vi "Alinhamento.vi"() -> ()   [LabVIEW 2019]
uses:
  <vilib>/silver_ctls/ArrayMatrixCluster/Real Matrix NI_Silver.ctl
panel:
  in  "MWU2987":i16
  in  "MWU2986":i16
  in  "MWU2985":i16
  in  "MWU2984":i16
  in  "MWU2983":i16
  in  "MWU2982":i16
  in  "MWU2981":i16
  in  "MWU2980":i16
  in  "MWU2979":i16
  in  "MWU2978":i16
  in  "MWU2977":i16
  in  "MWU2976":i16
  in  "MWU2975":i16
  in  "Tab Control":enum32{"Gráfico", "Matriz"}(tab)
  out "MWU1100":i16
  out "String lida em Caracter":string
  out "Gráfico":cluster{dbl, dbl, "Real Matrix":dbl[][]}(graph)
  out "Tubo":dbl(slide) scale=0.0..1950.0
  in  "Iniciar":bool
  in  "Parar":bool
  out "appended array":T1
  # "Valor enviado para a \ncomunicação"
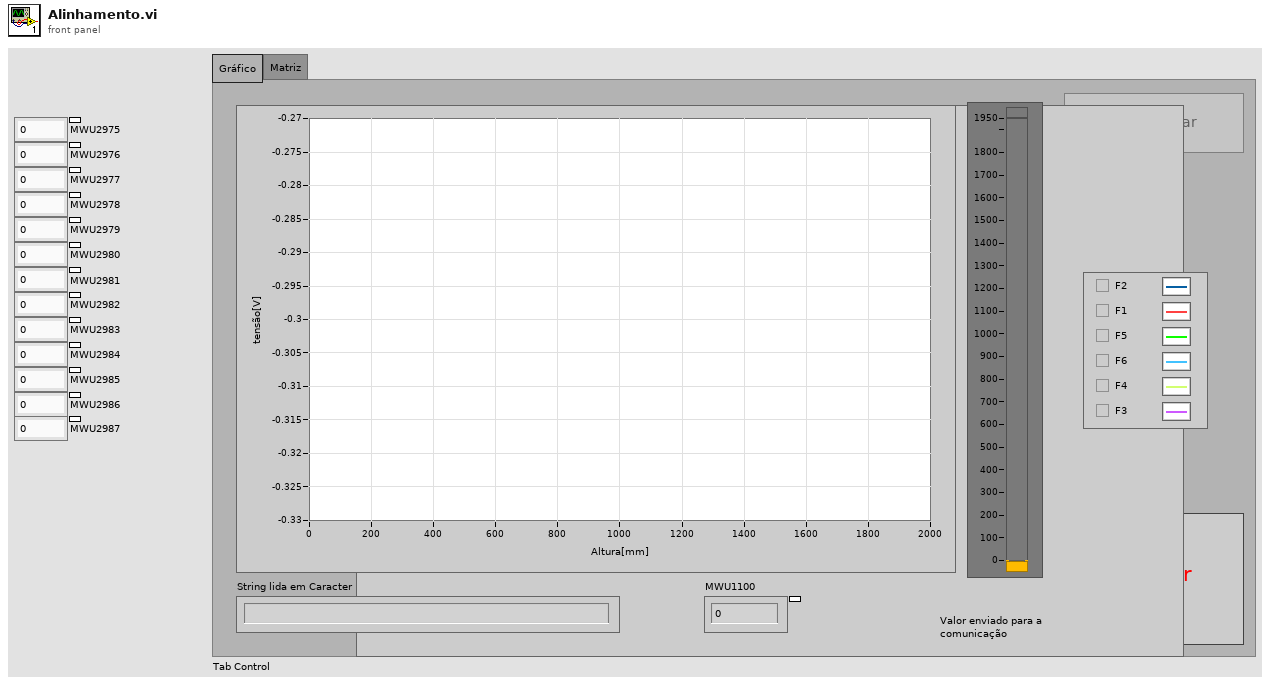
[diagram p1: front panel]
types:
  T1 = typedef "Real Matrix NI_Silver.ctl" = dbl[][]
  T2 = enum8{"Enabled", "Disabled", "Disabled and Grayed Out"}
  T3 = typedef "NI_Matrix.lvlib/RealMatrix.ctl" = dbl[][]
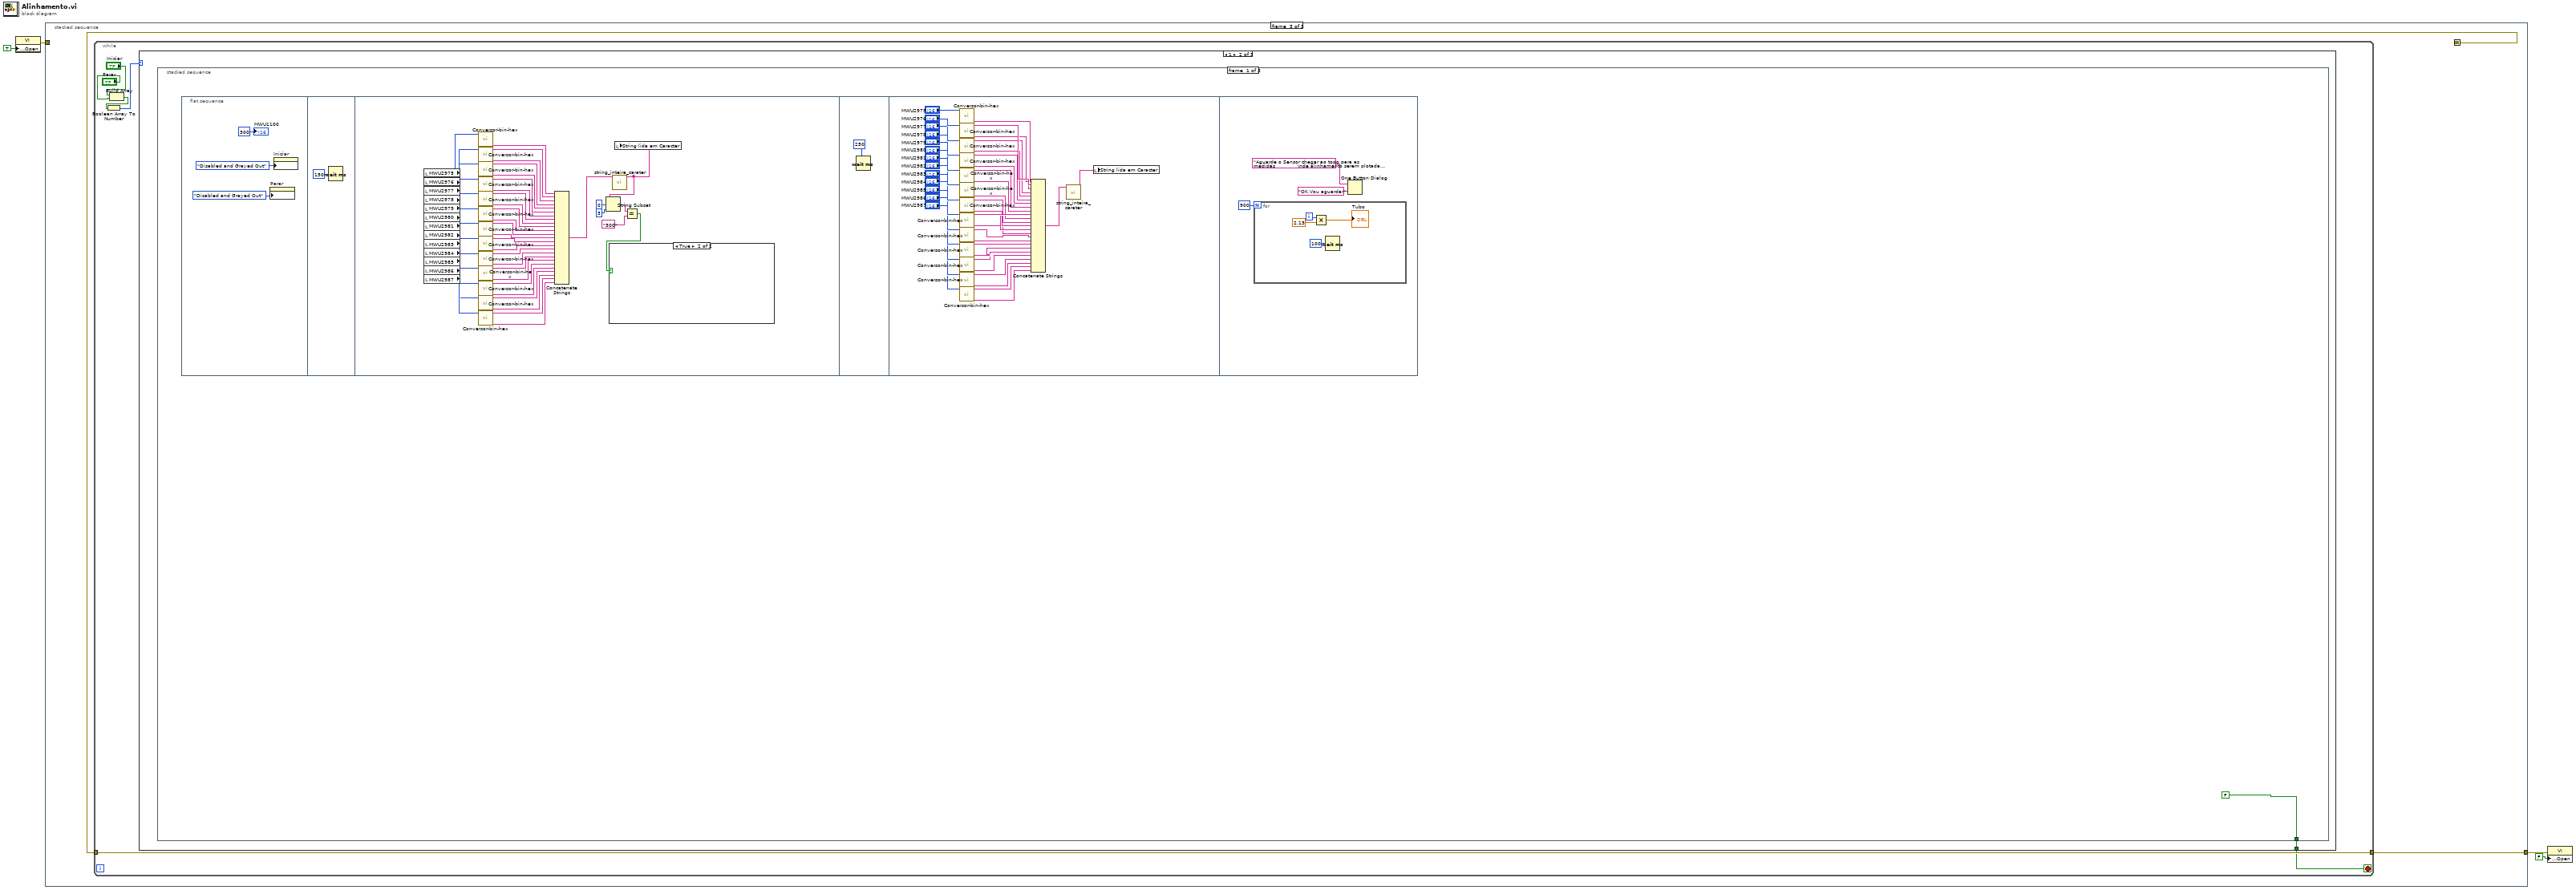
[diagram p0: block diagram]
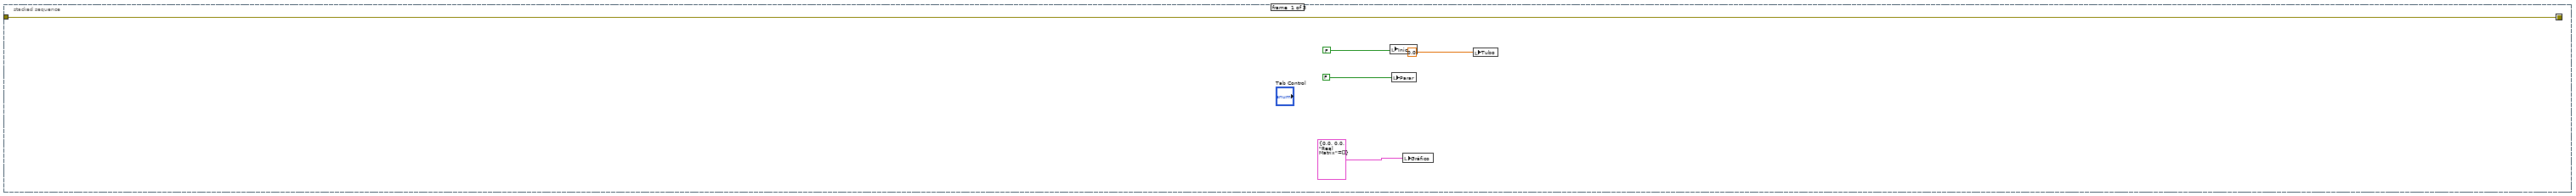
[diagram p2: hidden frame]
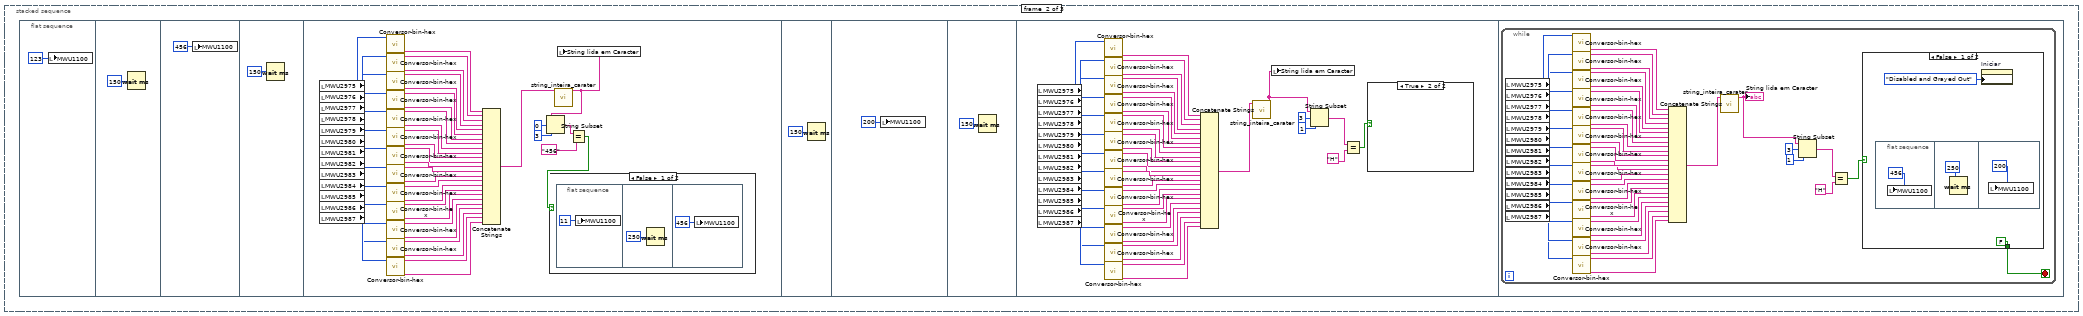
[diagram p3: hidden frame]
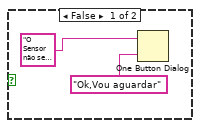
[diagram p5: hidden frame]
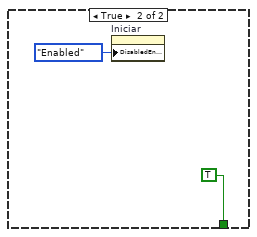
[diagram p6: hidden frame]
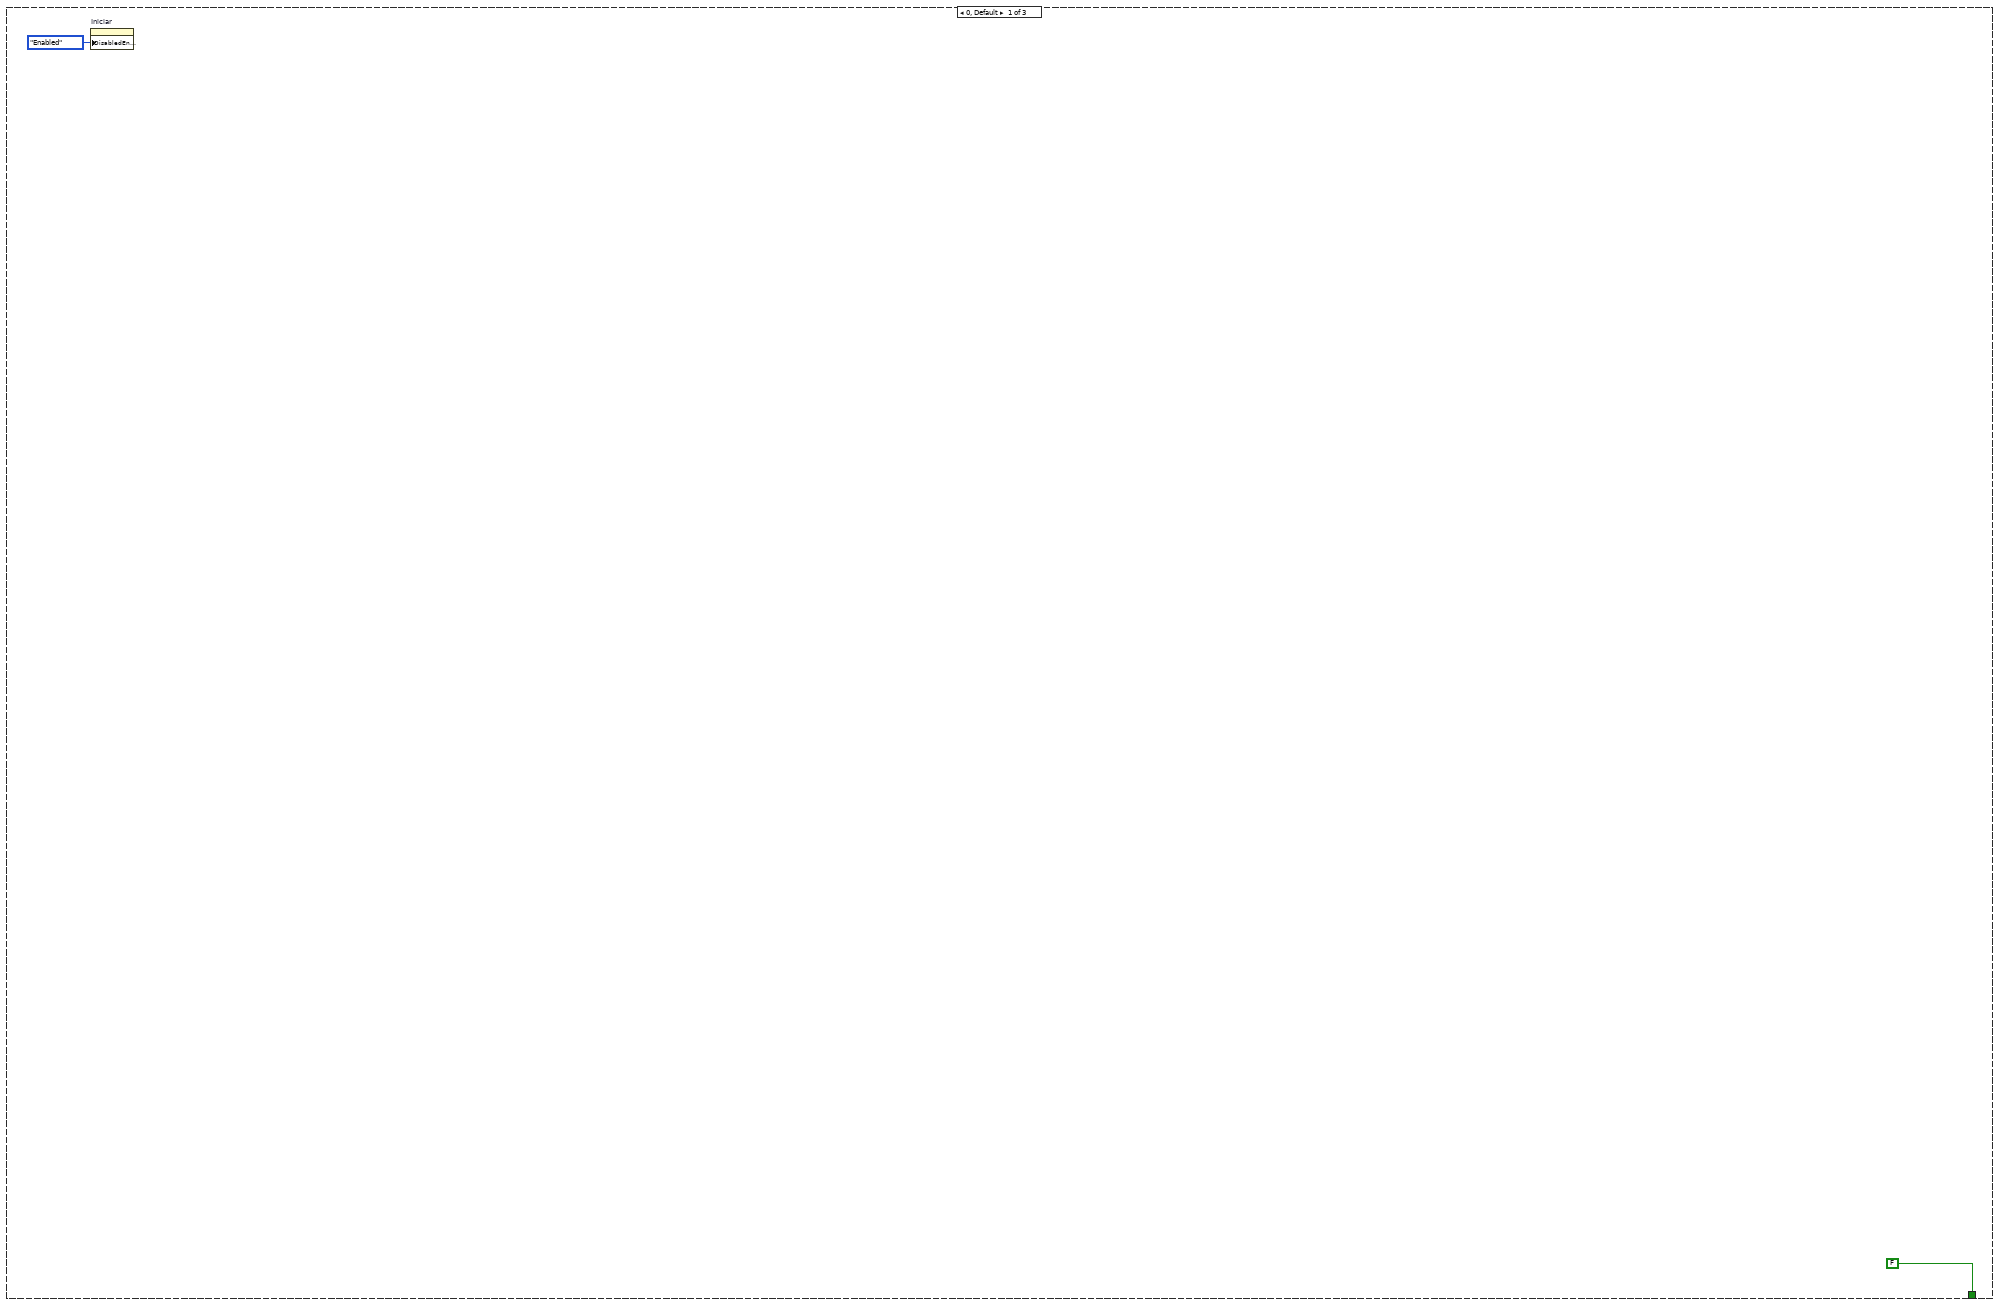
[diagram p7: hidden frame]
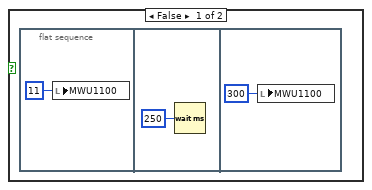
[diagram p8: hidden frame]
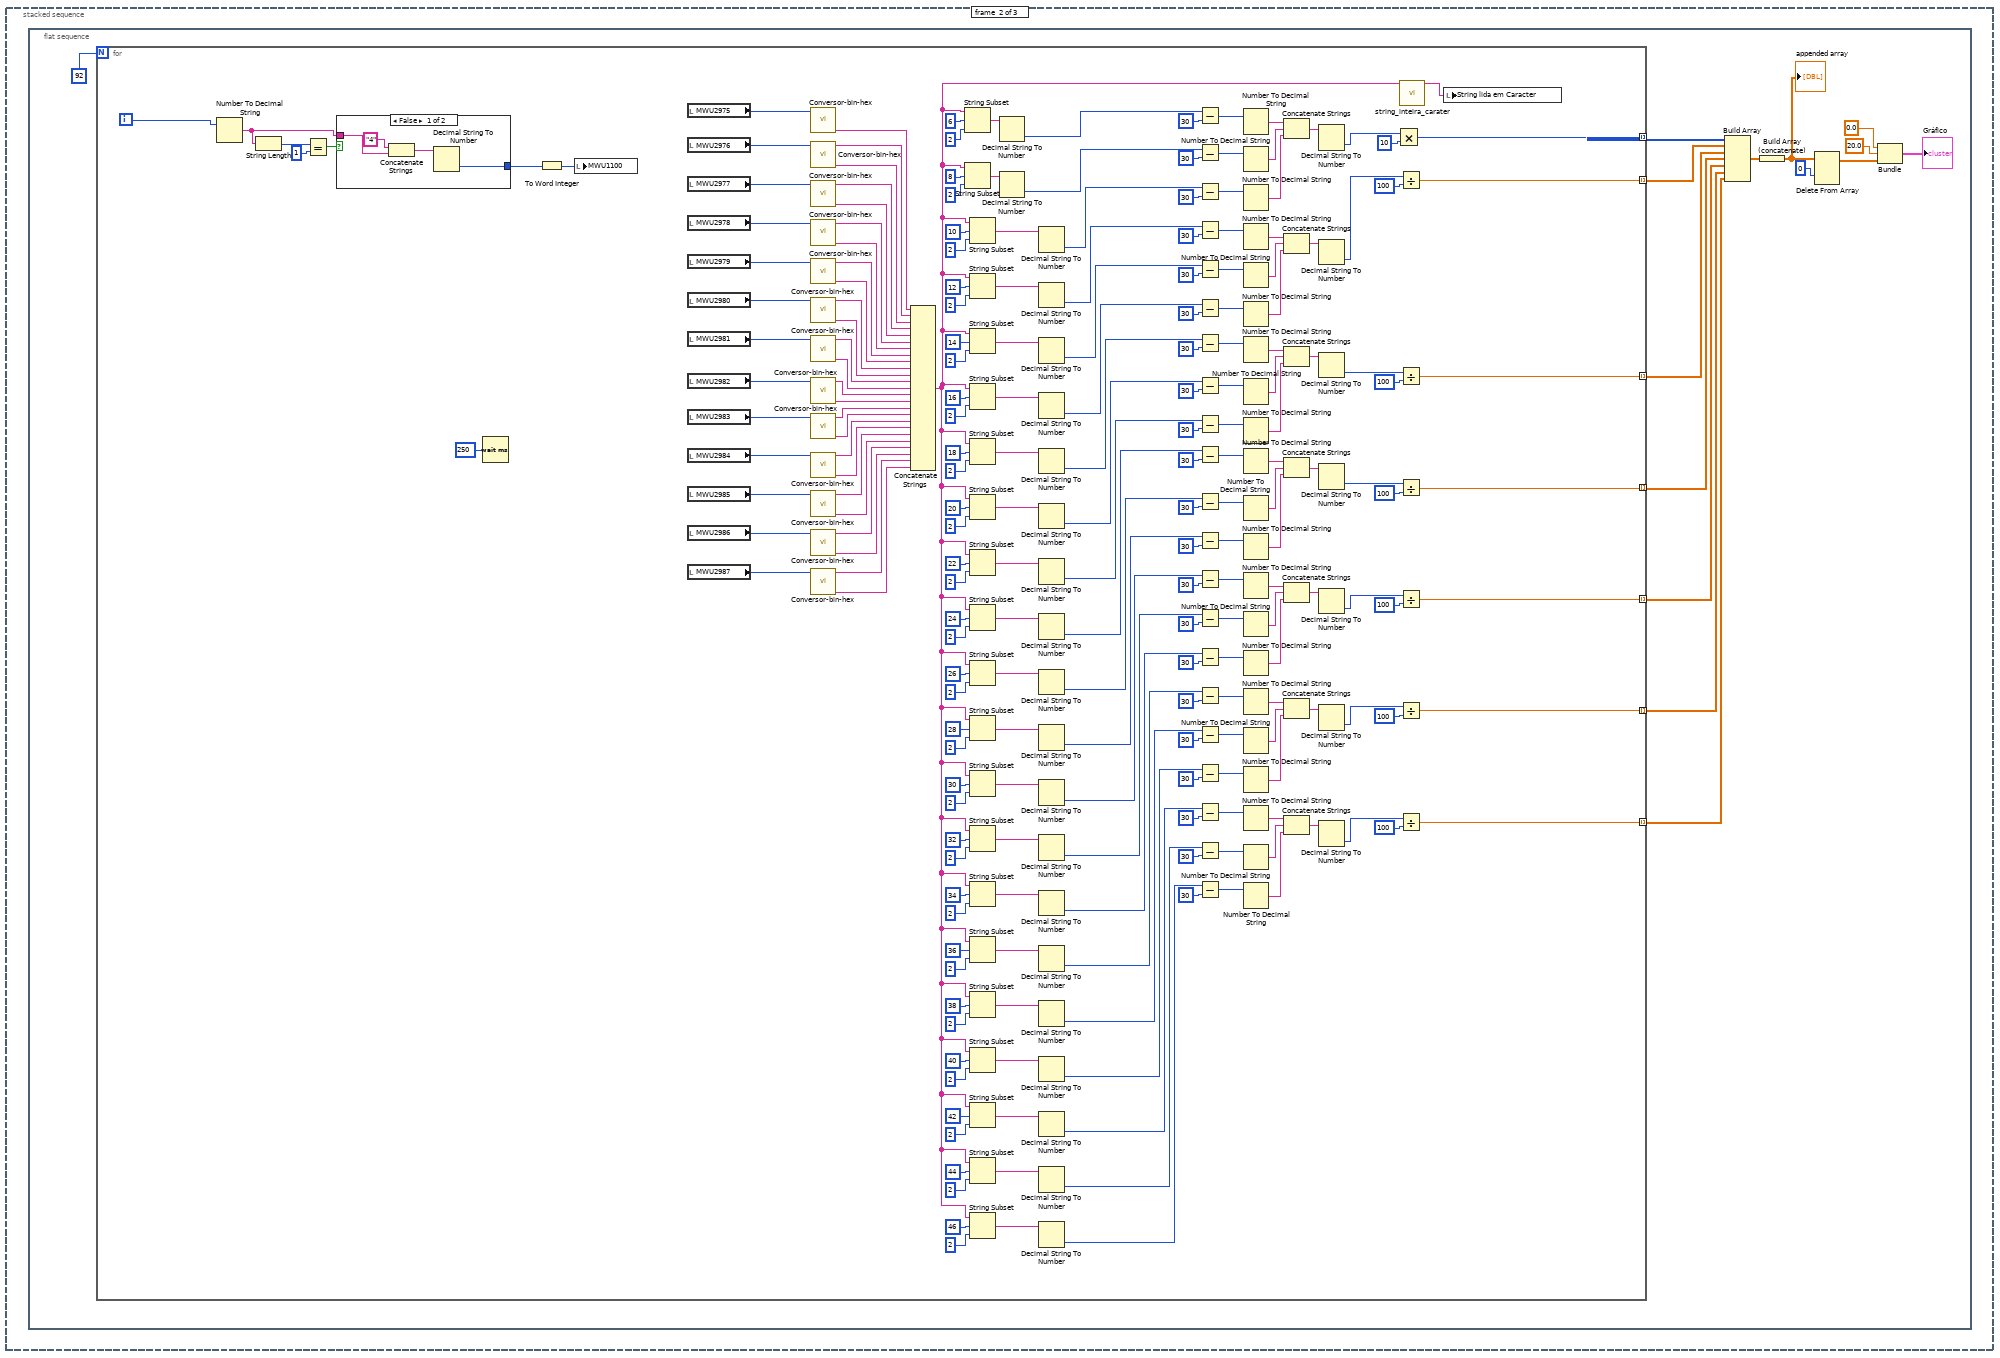
[diagram p9: hidden frame]
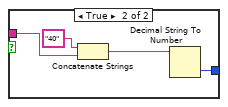
[diagram p10: hidden frame]
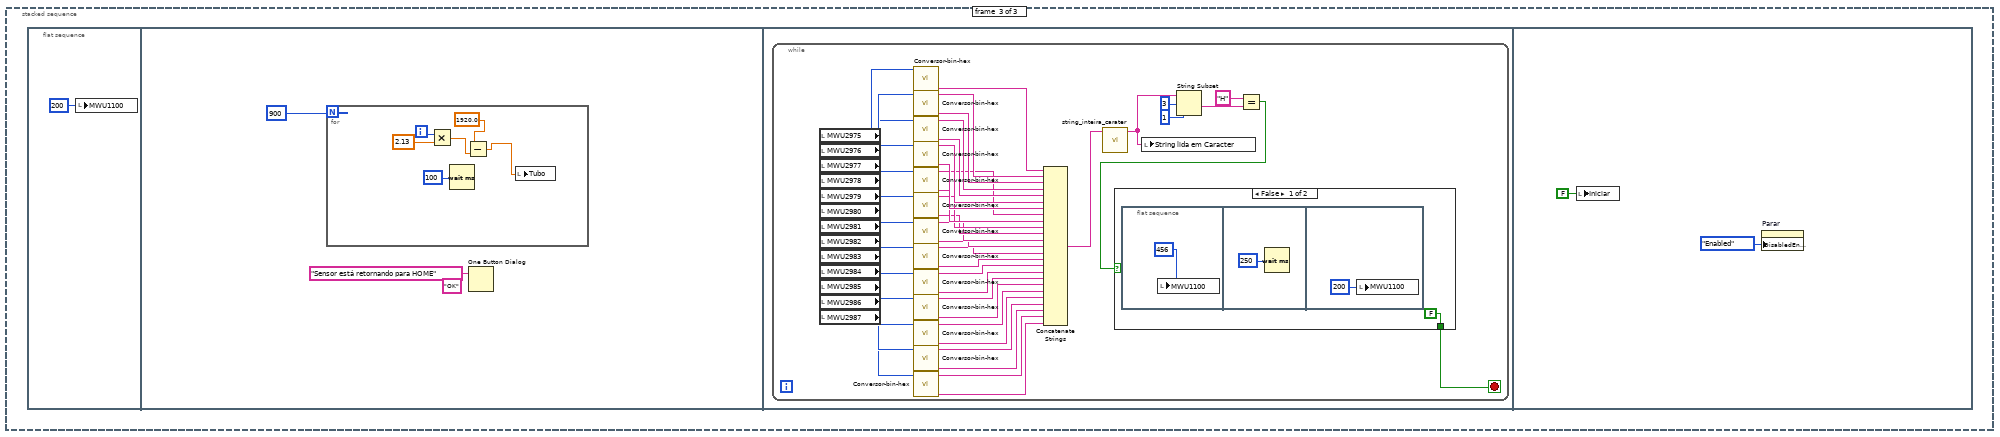
[diagram p11: hidden frame]
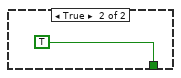
[diagram p12: hidden frame]
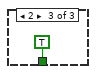
[diagram p13: hidden frame]
diagram:
  n1 = property class="VI"("Front Panel.Open"=TRUE ("Front Panel Window:Open")) -> (error out=w2:errorcluster)  [unwired: 2 in, 1 out]
  n2 = stacked-sequence {
    seq-local: [w9 _ _] -> [_ _ w166]
    tunnel: w2 -> [w9 _ _]
    tunnel: [_ _ w165] -> w1
    frame #0 {
      n3 = local write "Iniciar"(FALSE ("Iniciar")) -> ()
      n4 = local write "Parar"(FALSE ("Parar")) -> ()
      n5 = local write "Gráfico"(cluster{dbl, dbl, "Real Matrix":dbl[][]} {0.0, 0.0, "Real Matrix"=[]} ("Gráfico")) -> ()
      n6 = local write "Tubo"(0.0 ("Tubo")) -> ()
    }
    frame #1 {
      n7 = flat-sequence {
        frame #0 {
          n8 = local write "MWU1100"(i16 123 ("MWU1100")) -> ()
        }
        frame #1 {
          n9 = Wait (ms)(milliseconds to wait=u32 150) -> ()  [unwired: 1 out]
        }
        frame #2 {
          n10 = local write "MWU1100"(i16 456 ("MWU1100")) -> ()
        }
        frame #3 {
          n11 = Wait (ms)(milliseconds to wait=u32 150) -> ()  [unwired: 1 out]
        }
        frame #4 {
          n12 = local read "MWU2975"() -> (w44:i16)
          n13 = local read "MWU2976"() -> (w45:i16)
          n14 = local read "MWU2977"() -> (w46:i16)
          n15 = local read "MWU2978"() -> (w47:i16)
          n16 = local read "MWU2979"() -> (w48:i16)
          n17 = local read "MWU2980"() -> (w49:i16)
          n18 = local read "MWU2981"() -> (w50:i16)
          n19 = local read "MWU2982"() -> (w51:i16)
          n20 = local read "MWU2983"() -> (w52:i16)
          n21 = local read "MWU2984"() -> (w53:i16)
          n22 = local read "MWU2985"() -> (w54:i16)
          n23 = local read "MWU2986"() -> (w55:i16)
          n24 = local read "MWU2987"() -> (w56:i16)
          n25 = call "Conversor-bin-hex.vi"("Numeric"=w44) -> ("hex integer string"=w20:string)  [unwired: 9 in, 1 out]
          n26 = call "Conversor-bin-hex.vi"("Numeric"=w45) -> ("hex integer string"=w22:string, "hex integer string 2"=w21:string)  [unwired: 9 in]
          n27 = call "Conversor-bin-hex.vi"("Numeric"=w46) -> ("hex integer string"=w24:string, "hex integer string 2"=w23:string)  [unwired: 9 in]
          n28 = call "Conversor-bin-hex.vi"("Numeric"=w47) -> ("hex integer string"=w26:string, "hex integer string 2"=w25:string)  [unwired: 9 in]
          n29 = call "Conversor-bin-hex.vi"("Numeric"=w48) -> ("hex integer string"=w28:string, "hex integer string 2"=w27:string)  [unwired: 9 in]
          n30 = call "Conversor-bin-hex.vi"("Numeric"=w49) -> ("hex integer string"=w30:string, "hex integer string 2"=w29:string)  [unwired: 9 in]
          n31 = call "Conversor-bin-hex.vi"("Numeric"=w50) -> ("hex integer string"=w32:string, "hex integer string 2"=w31:string)  [unwired: 9 in]
          n32 = call "Conversor-bin-hex.vi"("Numeric"=w51) -> ("hex integer string"=w34:string, "hex integer string 2"=w33:string)  [unwired: 9 in]
          n33 = call "Conversor-bin-hex.vi"("Numeric"=w52) -> ("hex integer string"=w36:string, "hex integer string 2"=w35:string)  [unwired: 9 in]
          n34 = call "Conversor-bin-hex.vi"("Numeric"=w53) -> ("hex integer string"=w38:string, "hex integer string 2"=w37:string)  [unwired: 9 in]
          n35 = call "Conversor-bin-hex.vi"("Numeric"=w54) -> ("hex integer string"=w40:string, "hex integer string 2"=w39:string)  [unwired: 9 in]
          n36 = call "Conversor-bin-hex.vi"("Numeric"=w55) -> ("hex integer string"=w42:string, "hex integer string 2"=w41:string)  [unwired: 9 in]
          n37 = call "Conversor-bin-hex.vi"("Numeric"=w56) -> ("hex integer string"=w57:string, "hex integer string 2"=w43:string)  [unwired: 9 in]
          n38 = Concatenate Strings(w20, w21, w22, w23, w24, w25, w26, w27, w28, w29, w30, w31, w32, w33, w34, w35, w36, w37, w38, w39, w40, w41, w42, w43, w57) -> (w58:string)
          n39 = call "string_inteira_carater.vi"("String in"=w58) -> ("String out"=w19:string)  [unwired: 10 in]
          n40 = String Subset(string=w19, offset (0)=0, length (rest)=3 ("length (rest)")) -> (substring=w16:string)
          n41 = local write "String lida em Caracter"(w19) -> ()
          n42 = Equal?(x=w16, y="456") -> (x = y?=w14:bool)
          n43 = case shown="False" w14 {
            frame False {
              n44 = flat-sequence {
                frame #0 {
                  n45 = local write "MWU1100"(i16 11 ("MWU1100")) -> ()
                }
                frame #1 {
                  n46 = Wait (ms)(milliseconds to wait=u32 250) -> ()  [unwired: 1 out]
                }
                frame #2 {
                  n47 = local write "MWU1100"(i16 456 ("MWU1100")) -> ()
                }
              }
            }
            frame True {
            }
          }
        }
        frame #5 {
          n48 = Wait (ms)(milliseconds to wait=u32 150) -> ()  [unwired: 1 out]
        }
        frame #6 {
          n49 = local write "MWU1100"(i16 200 ("MWU1100")) -> ()
        }
        frame #7 {
          n50 = Wait (ms)(milliseconds to wait=u32 150) -> ()  [unwired: 1 out]
        }
        frame #8 {
          n51 = local read "MWU2975"() -> (w71:i16)
          n52 = local read "MWU2976"() -> (w96:i16)
          n53 = local read "MWU2977"() -> (w97:i16)
          n54 = local read "MWU2978"() -> (w98:i16)
          n55 = local read "MWU2979"() -> (w99:i16)
          n56 = local read "MWU2980"() -> (w100:i16)
          n57 = local read "MWU2981"() -> (w101:i16)
          n58 = local read "MWU2982"() -> (w102:i16)
          n59 = local read "MWU2983"() -> (w103:i16)
          n60 = local read "MWU2984"() -> (w104:i16)
          n61 = local read "MWU2985"() -> (w105:i16)
          n62 = local read "MWU2986"() -> (w106:i16)
          n63 = local read "MWU2987"() -> (w107:i16)
          n64 = call "Conversor-bin-hex.vi"("Numeric"=w71) -> ("hex integer string"=w72:string)  [unwired: 9 in, 1 out]
          n65 = call "Conversor-bin-hex.vi"("Numeric"=w96) -> ("hex integer string"=w74:string, "hex integer string 2"=w73:string)  [unwired: 9 in]
          n66 = call "Conversor-bin-hex.vi"("Numeric"=w97) -> ("hex integer string"=w76:string, "hex integer string 2"=w75:string)  [unwired: 9 in]
          n67 = call "Conversor-bin-hex.vi"("Numeric"=w98) -> ("hex integer string"=w78:string, "hex integer string 2"=w77:string)  [unwired: 9 in]
          n68 = call "Conversor-bin-hex.vi"("Numeric"=w99) -> ("hex integer string"=w80:string, "hex integer string 2"=w79:string)  [unwired: 9 in]
          n69 = call "Conversor-bin-hex.vi"("Numeric"=w100) -> ("hex integer string"=w82:string, "hex integer string 2"=w81:string)  [unwired: 9 in]
          n70 = call "Conversor-bin-hex.vi"("Numeric"=w101) -> ("hex integer string"=w84:string, "hex integer string 2"=w83:string)  [unwired: 9 in]
          n71 = call "Conversor-bin-hex.vi"("Numeric"=w102) -> ("hex integer string"=w86:string, "hex integer string 2"=w85:string)  [unwired: 9 in]
          n72 = call "Conversor-bin-hex.vi"("Numeric"=w103) -> ("hex integer string"=w88:string, "hex integer string 2"=w87:string)  [unwired: 9 in]
          n73 = call "Conversor-bin-hex.vi"("Numeric"=w104) -> ("hex integer string"=w90:string, "hex integer string 2"=w89:string)  [unwired: 9 in]
          n74 = call "Conversor-bin-hex.vi"("Numeric"=w105) -> ("hex integer string"=w92:string, "hex integer string 2"=w91:string)  [unwired: 9 in]
          n75 = call "Conversor-bin-hex.vi"("Numeric"=w106) -> ("hex integer string"=w94:string, "hex integer string 2"=w93:string)  [unwired: 9 in]
          n76 = call "Conversor-bin-hex.vi"("Numeric"=w107) -> ("hex integer string"=w108:string, "hex integer string 2"=w95:string)  [unwired: 9 in]
          n77 = Concatenate Strings(w72, w73, w74, w75, w76, w77, w78, w79, w80, w81, w82, w83, w84, w85, w86, w87, w88, w89, w90, w91, w92, w93, w94, w95, w108) -> (w109:string)
          n78 = call "string_inteira_carater.vi"("String in"=w109) -> ("String out"=w66:string)  [unwired: 10 in]
          n79 = local write "String lida em Caracter"(w66) -> ()
          n80 = String Subset(string=w66, offset (0)=3, length (rest)=1 ("length (rest)")) -> (substring=w67:string)
          n81 = Equal?(x=w67, y="H") -> (x = y?=w65:bool)
          n82 = case shown="True" w65 {
            frame False {
              n83 = One Button Dialog(message="O Sensor não se encontra em HOME                          \nEle já está descendo, aguarde chegar para começar o alinhamento", button name ("OK")="Ok,Vou aguardar") -> ()  [unwired: 1 out]
            }
            frame True {
            }
          }
        }
        frame #9 {
          n84 = while {
            stop <- w113 stop-if-true
            n85 = local read "MWU2975"() -> (w133:i16)
            n86 = local read "MWU2976"() -> (w132:i16)
            n87 = local read "MWU2977"() -> (w131:i16)
            n88 = local read "MWU2978"() -> (w130:i16)
            n89 = local read "MWU2979"() -> (w129:i16)
            n90 = local read "MWU2980"() -> (w128:i16)
            n91 = local read "MWU2981"() -> (w127:i16)
            n92 = local read "MWU2982"() -> (w126:i16)
            n93 = local read "MWU2983"() -> (w125:i16)
            n94 = local read "MWU2984"() -> (w124:i16)
            n95 = local read "MWU2985"() -> (w123:i16)
            n96 = local read "MWU2986"() -> (w122:i16)
            n97 = local read "MWU2987"() -> (w121:i16)
            n98 = call "Conversor-bin-hex.vi"("Numeric"=w133) -> ("hex integer string"=w157:string)  [unwired: 9 in, 1 out]
            n99 = call "Conversor-bin-hex.vi"("Numeric"=w132) -> ("hex integer string"=w155:string, "hex integer string 2"=w156:string)  [unwired: 9 in]
            n100 = call "Conversor-bin-hex.vi"("Numeric"=w131) -> ("hex integer string"=w153:string, "hex integer string 2"=w154:string)  [unwired: 9 in]
            n101 = call "Conversor-bin-hex.vi"("Numeric"=w130) -> ("hex integer string"=w151:string, "hex integer string 2"=w152:string)  [unwired: 9 in]
            n102 = call "Conversor-bin-hex.vi"("Numeric"=w129) -> ("hex integer string"=w149:string, "hex integer string 2"=w150:string)  [unwired: 9 in]
            n103 = call "Conversor-bin-hex.vi"("Numeric"=w128) -> ("hex integer string"=w147:string, "hex integer string 2"=w148:string)  [unwired: 9 in]
            n104 = call "Conversor-bin-hex.vi"("Numeric"=w127) -> ("hex integer string"=w145:string, "hex integer string 2"=w146:string)  [unwired: 9 in]
            n105 = call "Conversor-bin-hex.vi"("Numeric"=w126) -> ("hex integer string"=w143:string, "hex integer string 2"=w144:string)  [unwired: 9 in]
            n106 = call "Conversor-bin-hex.vi"("Numeric"=w125) -> ("hex integer string"=w141:string, "hex integer string 2"=w142:string)  [unwired: 9 in]
            n107 = call "Conversor-bin-hex.vi"("Numeric"=w124) -> ("hex integer string"=w139:string, "hex integer string 2"=w140:string)  [unwired: 9 in]
            n108 = call "Conversor-bin-hex.vi"("Numeric"=w123) -> ("hex integer string"=w137:string, "hex integer string 2"=w138:string)  [unwired: 9 in]
            n109 = call "Conversor-bin-hex.vi"("Numeric"=w122) -> ("hex integer string"=w135:string, "hex integer string 2"=w136:string)  [unwired: 9 in]
            n110 = call "Conversor-bin-hex.vi"("Numeric"=w121) -> ("hex integer string"=w120:string, "hex integer string 2"=w134:string)  [unwired: 9 in]
            n111 = Concatenate Strings(w157, w156, w155, w154, w153, w152, w151, w150, w149, w148, w147, w146, w145, w144, w143, w142, w141, w140, w139, w138, w137, w136, w135, w134, w120) -> (w115:string)
            n112 = call "string_inteira_carater.vi"("String in"=w115) -> ("String out"=w114:string)  [unwired: 10 in]
            "String lida em Caracter" <- w114
            n113 = String Subset(string=w114, offset (0)=3, length (rest)=1 ("length (rest)")) -> (substring=w116:string)
            n114 = Equal?(x=w116, y="H") -> (x = y?=w112:bool)
            n115 = case shown="False" w112 {
              tunnel: [FALSE TRUE] -> w113
              frame False {
                n116 = flat-sequence {
                  frame #0 {
                    n117 = local write "MWU1100"(i16 456 ("MWU1100")) -> ()
                  }
                  frame #1 {
                    n118 = Wait (ms)(milliseconds to wait=u32 250) -> ()  [unwired: 1 out]
                  }
                  frame #2 {
                    n119 = local write "MWU1100"(i16 200 ("MWU1100")) -> ()
                  }
                }
                n120 = property on="Iniciar" class="Bool (strict)"("DisabledEnum"=T2."Disabled and Grayed Out" ("Disabled")) -> ()  [unwired: 2 in, 2 out]
              }
              frame True {
                n121 = property on="Iniciar" class="Bool (strict)"("DisabledEnum"=T2."Enabled" ("Disabled")) -> ()  [unwired: 2 in, 2 out]
              }
            }
          }
        }
      }
    }
    frame #2 {
      n122 = while {
        tunnel: w166 -> [w172]
        tunnel: [w172] -> w165
        stop <- w168 stop-if-true
        n123 = Build Array("Iniciar", "Parar") -> (w170:bool[])
        n124 = Boolean Array To Number(Boolean array=w170) -> (number=w169:u32)
        n125 = case shown="1" w169 {
          tunnel: [FALSE w175 TRUE] -> w168
          frame 0, Default {
            n126 = property on="Iniciar" class="Bool (strict)"("DisabledEnum"=T2."Enabled" ("Disabled")) -> ()  [unwired: 2 in, 2 out]
          }
          frame 1 {
            n127 = stacked-sequence {
              tunnel: [FALSE _ _] -> w175
              frame #0 {
                n128 = flat-sequence {
                  frame #0 {
                    n129 = property on="Parar" class="Bool (strict)"("DisabledEnum"=T2."Disabled and Grayed Out" ("Disabled")) -> ()  [unwired: 2 in, 2 out]
                    n130 = property on="Iniciar" class="Bool (strict)"("DisabledEnum"=T2."Disabled and Grayed Out" ("Disabled")) -> ()  [unwired: 2 in, 2 out]
                    "MWU1100" <- i16 300 ("MWU1100")
                  }
                  frame #1 {
                    n131 = Wait (ms)(milliseconds to wait=u32 150) -> ()  [unwired: 1 out]
                  }
                  frame #2 {
                    n132 = local read "MWU2975"() -> (w211:i16)
                    n133 = local read "MWU2976"() -> (w212:i16)
                    n134 = local read "MWU2977"() -> (w213:i16)
                    n135 = local read "MWU2978"() -> (w214:i16)
                    n136 = local read "MWU2979"() -> (w215:i16)
                    n137 = local read "MWU2980"() -> (w216:i16)
                    n138 = local read "MWU2981"() -> (w217:i16)
                    n139 = local read "MWU2982"() -> (w218:i16)
                    n140 = local read "MWU2983"() -> (w219:i16)
                    n141 = local read "MWU2984"() -> (w220:i16)
                    n142 = local read "MWU2985"() -> (w221:i16)
                    n143 = local read "MWU2986"() -> (w222:i16)
                    n144 = local read "MWU2987"() -> (w223:i16)
                    n145 = call "Conversor-bin-hex.vi"("Numeric"=w211) -> ("hex integer string"=w187:string)  [unwired: 9 in, 1 out]
                    n146 = call "Conversor-bin-hex.vi"("Numeric"=w212) -> ("hex integer string"=w189:string, "hex integer string 2"=w188:string)  [unwired: 9 in]
                    n147 = call "Conversor-bin-hex.vi"("Numeric"=w213) -> ("hex integer string"=w191:string, "hex integer string 2"=w190:string)  [unwired: 9 in]
                    n148 = call "Conversor-bin-hex.vi"("Numeric"=w214) -> ("hex integer string"=w193:string, "hex integer string 2"=w192:string)  [unwired: 9 in]
                    n149 = call "Conversor-bin-hex.vi"("Numeric"=w215) -> ("hex integer string"=w195:string, "hex integer string 2"=w194:string)  [unwired: 9 in]
                    n150 = call "Conversor-bin-hex.vi"("Numeric"=w216) -> ("hex integer string"=w197:string, "hex integer string 2"=w196:string)  [unwired: 9 in]
                    n151 = call "Conversor-bin-hex.vi"("Numeric"=w217) -> ("hex integer string"=w199:string, "hex integer string 2"=w198:string)  [unwired: 9 in]
                    n152 = call "Conversor-bin-hex.vi"("Numeric"=w218) -> ("hex integer string"=w201:string, "hex integer string 2"=w200:string)  [unwired: 9 in]
                    n153 = call "Conversor-bin-hex.vi"("Numeric"=w219) -> ("hex integer string"=w203:string, "hex integer string 2"=w202:string)  [unwired: 9 in]
                    n154 = call "Conversor-bin-hex.vi"("Numeric"=w220) -> ("hex integer string"=w205:string, "hex integer string 2"=w204:string)  [unwired: 9 in]
                    n155 = call "Conversor-bin-hex.vi"("Numeric"=w221) -> ("hex integer string"=w207:string, "hex integer string 2"=w206:string)  [unwired: 9 in]
                    n156 = call "Conversor-bin-hex.vi"("Numeric"=w222) -> ("hex integer string"=w209:string, "hex integer string 2"=w208:string)  [unwired: 9 in]
                    n157 = call "Conversor-bin-hex.vi"("Numeric"=w223) -> ("hex integer string"=w224:string, "hex integer string 2"=w210:string)  [unwired: 9 in]
                    n158 = Concatenate Strings(w187, w188, w189, w190, w191, w192, w193, w194, w195, w196, w197, w198, w199, w200, w201, w202, w203, w204, w205, w206, w207, w208, w209, w210, w224) -> (w225:string)
                    n159 = call "string_inteira_carater.vi"("String in"=w225) -> ("String out"=w186:string)  [unwired: 10 in]
                    n160 = String Subset(string=w186, offset (0)=0, length (rest)=3 ("length (rest)")) -> (substring=w185:string)
                    n161 = local write "String lida em Caracter"(w186) -> ()
                    n162 = Equal?(x=w185, y="300") -> (x = y?=w184:bool)
                    n163 = case shown="True" w184 {
                      frame False {
                        n164 = flat-sequence {
                          frame #0 {
                            n165 = local write "MWU1100"(i16 11 ("MWU1100")) -> ()
                          }
                          frame #1 {
                            n166 = Wait (ms)(milliseconds to wait=u32 250) -> ()  [unwired: 1 out]
                          }
                          frame #2 {
                            n167 = local write "MWU1100"(i16 300 ("MWU1100")) -> ()
                          }
                        }
                      }
                      frame True {
                      }
                    }
                  }
                  frame #3 {
                    n168 = Wait (ms)(milliseconds to wait=u32 250) -> ()  [unwired: 1 out]
                  }
                  frame #4 {
                    n169 = call "Conversor-bin-hex.vi"("Numeric"="MWU2975") -> ("hex integer string"=w269:string)  [unwired: 9 in, 1 out]
                    n170 = call "Conversor-bin-hex.vi"("Numeric"="MWU2976") -> ("hex integer string"=w267:string, "hex integer string 2"=w268:string)  [unwired: 9 in]
                    n171 = call "Conversor-bin-hex.vi"("Numeric"="MWU2977") -> ("hex integer string"=w265:string, "hex integer string 2"=w266:string)  [unwired: 9 in]
                    n172 = call "Conversor-bin-hex.vi"("Numeric"="MWU2978") -> ("hex integer string"=w263:string, "hex integer string 2"=w264:string)  [unwired: 9 in]
                    n173 = call "Conversor-bin-hex.vi"("Numeric"="MWU2979") -> ("hex integer string"=w261:string, "hex integer string 2"=w262:string)  [unwired: 9 in]
                    n174 = call "Conversor-bin-hex.vi"("Numeric"="MWU2980") -> ("hex integer string"=w259:string, "hex integer string 2"=w260:string)  [unwired: 9 in]
                    n175 = call "Conversor-bin-hex.vi"("Numeric"="MWU2981") -> ("hex integer string"=w257:string, "hex integer string 2"=w258:string)  [unwired: 9 in]
                    n176 = call "Conversor-bin-hex.vi"("Numeric"="MWU2982") -> ("hex integer string"=w255:string, "hex integer string 2"=w256:string)  [unwired: 9 in]
                    n177 = call "Conversor-bin-hex.vi"("Numeric"="MWU2983") -> ("hex integer string"=w253:string, "hex integer string 2"=w254:string)  [unwired: 9 in]
                    n178 = call "Conversor-bin-hex.vi"("Numeric"="MWU2984") -> ("hex integer string"=w251:string, "hex integer string 2"=w252:string)  [unwired: 9 in]
                    n179 = call "Conversor-bin-hex.vi"("Numeric"="MWU2985") -> ("hex integer string"=w249:string, "hex integer string 2"=w250:string)  [unwired: 9 in]
                    n180 = call "Conversor-bin-hex.vi"("Numeric"="MWU2986") -> ("hex integer string"=w247:string, "hex integer string 2"=w248:string)  [unwired: 9 in]
                    n181 = call "Conversor-bin-hex.vi"("Numeric"="MWU2987") -> ("hex integer string"=w232:string, "hex integer string 2"=w246:string)  [unwired: 9 in]
                    n182 = Concatenate Strings(w269, w268, w267, w266, w265, w264, w263, w262, w261, w260, w259, w258, w257, w256, w255, w254, w253, w252, w251, w250, w249, w248, w247, w246, w232) -> (w231:string)
                    n183 = call "string_inteira_carater.vi"("String in"=w231) -> ("String out"=w230:string)  [unwired: 10 in]
                    n184 = local write "String lida em Caracter"(w230) -> ()
                  }
                  frame #5 {
                    n185 = for {
                      N: 900 -> [_]
                      i -> [w275]
                      n186 = Multiply(x=w275, y=2.13) -> (x*y=→"Tubo":dbl)
                      n187 = Wait (ms)(milliseconds to wait=u32 100) -> ()  [unwired: 1 out]
                    }
                    n188 = One Button Dialog(message="Aguarde o Sensor chegar ao topo para as medidas              \nde alinhamento serem plotadas no gráfico                    \nleva cerca de 1 minuto e meio, acompanhe o percurso pelo display vertical", button name ("OK")="OK,Vou aguardar") -> ()  [unwired: 1 out]
                  }
                }
              }
              frame #1 {
                n189 = flat-sequence {
                  frame #0 {
                    n190 = for {
                      N: 92 -> [_]
                      tunnel: [w504] -> w285 mode=indexing
                      tunnel: [w511] -> w291 mode=indexing
                      tunnel: [w502] -> w286 mode=indexing
                      tunnel: [w500] -> w287 mode=indexing
                      tunnel: [w497] -> w288 mode=indexing
                      tunnel: [w495] -> w289 mode=indexing
                      tunnel: [w493] -> w290 mode=indexing
                      i -> [w514]
                      n191 = Number To Decimal String(number=w514) -> (decimal integer string=w298:string)  [unwired: 1 in]
                      n192 = String Length(string=w298) -> (length=w301:i32)
                      n193 = Equal?(x=w301, y=1) -> (x = y?=w299:bool)
                      n194 = case shown="False" w299 {
                        tunnel: w298 -> [w517 w521]
                        tunnel: [w515 w519] -> w296
                        frame False {
                          n195 = Concatenate Strings("4" ("string"), w517) -> (w516:string)
                          n196 = Decimal String To Number(string=w516) -> (number=w515:i32)  [unwired: 2 in, 1 out]
                        }
                        frame True {
                          n197 = Concatenate Strings("40" ("string"), w521) -> (w520:string)
                          n198 = Decimal String To Number(string=w520) -> (number=w519:i32)  [unwired: 2 in, 1 out]
                        }
                      }
                      n199 = Wait (ms)(milliseconds to wait=u32 250) -> ()  [unwired: 1 out]
                      n200 = To Word Integer(number=w296) -> (16bit integer=w297:i16)
                      n201 = local write "MWU1100"(w297) -> ()
                      n202 = local read "MWU2975"() -> (w314:i16)
                      n203 = local read "MWU2976"() -> (w313:i16)
                      n204 = local read "MWU2977"() -> (w312:i16)
                      n205 = local read "MWU2978"() -> (w311:i16)
                      n206 = local read "MWU2979"() -> (w310:i16)
                      n207 = local read "MWU2980"() -> (w309:i16)
                      n208 = local read "MWU2981"() -> (w308:i16)
                      n209 = local read "MWU2982"() -> (w307:i16)
                      n210 = local read "MWU2983"() -> (w306:i16)
                      n211 = local read "MWU2984"() -> (w305:i16)
                      n212 = local read "MWU2985"() -> (w304:i16)
                      n213 = local read "MWU2986"() -> (w303:i16)
                      n214 = local read "MWU2987"() -> (w302:i16)
                      n215 = call "Conversor-bin-hex.vi"("Numeric"=w314) -> ("hex integer string"=w491:string)  [unwired: 9 in, 1 out]
                      n216 = call "Conversor-bin-hex.vi"("Numeric"=w313) -> ("hex integer string"=w489:string, "hex integer string 2"=w490:string)  [unwired: 9 in]
                      n217 = call "Conversor-bin-hex.vi"("Numeric"=w312) -> ("hex integer string"=w487:string, "hex integer string 2"=w488:string)  [unwired: 9 in]
                      n218 = call "Conversor-bin-hex.vi"("Numeric"=w311) -> ("hex integer string"=w485:string, "hex integer string 2"=w486:string)  [unwired: 9 in]
                      n219 = call "Conversor-bin-hex.vi"("Numeric"=w310) -> ("hex integer string"=w483:string, "hex integer string 2"=w484:string)  [unwired: 9 in]
                      n220 = call "Conversor-bin-hex.vi"("Numeric"=w309) -> ("hex integer string"=w481:string, "hex integer string 2"=w482:string)  [unwired: 9 in]
                      n221 = call "Conversor-bin-hex.vi"("Numeric"=w308) -> ("hex integer string"=w479:string, "hex integer string 2"=w480:string)  [unwired: 9 in]
                      n222 = call "Conversor-bin-hex.vi"("Numeric"=w307) -> ("hex integer string"=w477:string, "hex integer string 2"=w478:string)  [unwired: 9 in]
                      n223 = call "Conversor-bin-hex.vi"("Numeric"=w306) -> ("hex integer string"=w475:string, "hex integer string 2"=w476:string)  [unwired: 9 in]
                      n224 = call "Conversor-bin-hex.vi"("Numeric"=w305) -> ("hex integer string"=w473:string, "hex integer string 2"=w474:string)  [unwired: 9 in]
                      n225 = call "Conversor-bin-hex.vi"("Numeric"=w304) -> ("hex integer string"=w471:string, "hex integer string 2"=w472:string)  [unwired: 9 in]
                      n226 = call "Conversor-bin-hex.vi"("Numeric"=w303) -> ("hex integer string"=w469:string, "hex integer string 2"=w470:string)  [unwired: 9 in]
                      n227 = call "Conversor-bin-hex.vi"("Numeric"=w302) -> ("hex integer string"=w294:string, "hex integer string 2"=w468:string)  [unwired: 9 in]
                      n228 = Concatenate Strings(w491, w490, w489, w488, w487, w486, w485, w484, w483, w482, w481, w480, w479, w478, w477, w476, w475, w474, w473, w472, w471, w470, w469, w468, w294) -> (w293:string)
                      n229 = String Subset(string=w293, offset (0)=6, length (rest)=2 ("length (rest)")) -> (substring=w318:string)
                      n230 = String Subset(string=w293, offset (0)=8, length (rest)=2 ("length (rest)")) -> (substring=w462:string)
                      n231 = String Subset(string=w293, offset (0)=10, length (rest)=2 ("length (rest)")) -> (substring=w463:string)
                      n232 = String Subset(string=w293, offset (0)=12, length (rest)=2 ("length (rest)")) -> (substring=w425:string)
                      n233 = String Subset(string=w293, offset (0)=14, length (rest)=2 ("length (rest)")) -> (substring=w431:string)
                      n234 = String Subset(string=w293, offset (0)=16, length (rest)=2 ("length (rest)")) -> (substring=w430:string)
                      n235 = String Subset(string=w293, offset (0)=18, length (rest)=2 ("length (rest)")) -> (substring=w424:string)
                      n236 = String Subset(string=w293, offset (0)=20, length (rest)=2 ("length (rest)")) -> (substring=w419:string)
                      n237 = String Subset(string=w293, offset (0)=22, length (rest)=2 ("length (rest)")) -> (substring=w420:string)
                      n238 = String Subset(string=w293, offset (0)=24, length (rest)=2 ("length (rest)")) -> (substring=w382:string)
                      n239 = String Subset(string=w293, offset (0)=26, length (rest)=2 ("length (rest)")) -> (substring=w388:string)
                      n240 = String Subset(string=w293, offset (0)=28, length (rest)=2 ("length (rest)")) -> (substring=w387:string)
                      n241 = String Subset(string=w293, offset (0)=30, length (rest)=2 ("length (rest)")) -> (substring=w381:string)
                      n242 = String Subset(string=w293, offset (0)=32, length (rest)=2 ("length (rest)")) -> (substring=w375:string)
                      n243 = String Subset(string=w293, offset (0)=34, length (rest)=2 ("length (rest)")) -> (substring=w376:string)
                      n244 = String Subset(string=w293, offset (0)=36, length (rest)=2 ("length (rest)")) -> (substring=w338:string)
                      n245 = String Subset(string=w293, offset (0)=38, length (rest)=2 ("length (rest)")) -> (substring=w344:string)
                      n246 = String Subset(string=w293, offset (0)=40, length (rest)=2 ("length (rest)")) -> (substring=w343:string)
                      n247 = String Subset(string=w293, offset (0)=42, length (rest)=2 ("length (rest)")) -> (substring=w320:string)
                      n248 = String Subset(string=w293, offset (0)=44, length (rest)=2 ("length (rest)")) -> (substring=w334:string)
                      n249 = String Subset(string=w293, offset (0)=46, length (rest)=2 ("length (rest)")) -> (substring=w335:string)
                      n250 = Decimal String To Number(string=w318) -> (number=w457:i32)  [unwired: 2 in, 1 out]
                      n251 = Decimal String To Number(string=w462) -> (number=w453:i32)  [unwired: 2 in, 1 out]
                      n252 = Decimal String To Number(string=w463) -> (number=w452:i32)  [unwired: 2 in, 1 out]
                      n253 = Decimal String To Number(string=w425) -> (number=w436:i32)  [unwired: 2 in, 1 out]
                      n254 = Decimal String To Number(string=w431) -> (number=w440:i32)  [unwired: 2 in, 1 out]
                      n255 = Decimal String To Number(string=w430) -> (number=w441:i32)  [unwired: 2 in, 1 out]
                      n256 = Decimal String To Number(string=w424) -> (number=w414:i32)  [unwired: 2 in, 1 out]
                      n257 = Decimal String To Number(string=w419) -> (number=w410:i32)  [unwired: 2 in, 1 out]
                      n258 = Decimal String To Number(string=w420) -> (number=w409:i32)  [unwired: 2 in, 1 out]
                      n259 = Decimal String To Number(string=w382) -> (number=w393:i32)  [unwired: 2 in, 1 out]
                      n260 = Decimal String To Number(string=w388) -> (number=w397:i32)  [unwired: 2 in, 1 out]
                      n261 = Decimal String To Number(string=w387) -> (number=w398:i32)  [unwired: 2 in, 1 out]
                      n262 = Decimal String To Number(string=w381) -> (number=w370:i32)  [unwired: 2 in, 1 out]
                      n263 = Decimal String To Number(string=w375) -> (number=w366:i32)  [unwired: 2 in, 1 out]
                      n264 = Decimal String To Number(string=w376) -> (number=w365:i32)  [unwired: 2 in, 1 out]
                      n265 = Decimal String To Number(string=w338) -> (number=w349:i32)  [unwired: 2 in, 1 out]
                      n266 = Decimal String To Number(string=w344) -> (number=w353:i32)  [unwired: 2 in, 1 out]
                      n267 = Decimal String To Number(string=w343) -> (number=w354:i32)  [unwired: 2 in, 1 out]
                      n268 = Decimal String To Number(string=w320) -> (number=w330:i32)  [unwired: 2 in, 1 out]
                      n269 = Decimal String To Number(string=w334) -> (number=w327:i32)  [unwired: 2 in, 1 out]
                      n270 = Decimal String To Number(string=w335) -> (number=w326:i32)  [unwired: 2 in, 1 out]
                      n271 = Subtract(x=w457, y=30) -> (x-y=w451:i32)
                      n272 = Subtract(x=w453, y=30) -> (x-y=w450:i32)
                      n273 = Subtract(x=w452, y=30) -> (x-y=w449:i32)
                      n274 = Subtract(x=w436, y=30) -> (x-y=w442:i32)
                      n275 = Subtract(x=w440, y=30) -> (x-y=w443:i32)
                      n276 = Subtract(x=w441, y=30) -> (x-y=w444:i32)
                      n277 = Subtract(x=w414, y=30) -> (x-y=w408:i32)
                      n278 = Subtract(x=w410, y=30) -> (x-y=w407:i32)
                      n279 = Subtract(x=w409, y=30) -> (x-y=w406:i32)
                      n280 = Subtract(x=w393, y=30) -> (x-y=w399:i32)
                      n281 = Subtract(x=w397, y=30) -> (x-y=w400:i32)
                      n282 = Subtract(x=w398, y=30) -> (x-y=w401:i32)
                      n283 = Subtract(x=w370, y=30) -> (x-y=w364:i32)
                      n284 = Subtract(x=w366, y=30) -> (x-y=w363:i32)
                      n285 = Subtract(x=w365, y=30) -> (x-y=w362:i32)
                      n286 = Subtract(x=w349, y=30) -> (x-y=w355:i32)
                      n287 = Subtract(x=w353, y=30) -> (x-y=w356:i32)
                      n288 = Subtract(x=w354, y=30) -> (x-y=w357:i32)
                      n289 = Subtract(x=w330, y=30) -> (x-y=w325:i32)
                      n290 = Subtract(x=w327, y=30) -> (x-y=w324:i32)
                      n291 = Subtract(x=w326, y=30) -> (x-y=w323:i32)
                      n292 = Number To Decimal String(number=w451) -> (decimal integer string=w461:string)  [unwired: 1 in]
                      n293 = Number To Decimal String(number=w450) -> (decimal integer string=w460:string)  [unwired: 1 in]
                      n294 = Number To Decimal String(number=w449) -> (decimal integer string=w459:string)  [unwired: 1 in]
                      n295 = Number To Decimal String(number=w442) -> (decimal integer string=w432:string)  [unwired: 1 in]
                      n296 = Number To Decimal String(number=w443) -> (decimal integer string=w433:string)  [unwired: 1 in]
                      n297 = Number To Decimal String(number=w444) -> (decimal integer string=w434:string)  [unwired: 1 in]
                      n298 = Number To Decimal String(number=w408) -> (decimal integer string=w418:string)  [unwired: 1 in]
                      n299 = Number To Decimal String(number=w407) -> (decimal integer string=w417:string)  [unwired: 1 in]
                      n300 = Number To Decimal String(number=w406) -> (decimal integer string=w416:string)  [unwired: 1 in]
                      n301 = Number To Decimal String(number=w399) -> (decimal integer string=w389:string)  [unwired: 1 in]
                      n302 = Number To Decimal String(number=w400) -> (decimal integer string=w390:string)  [unwired: 1 in]
                      n303 = Number To Decimal String(number=w401) -> (decimal integer string=w391:string)  [unwired: 1 in]
                      n304 = Number To Decimal String(number=w364) -> (decimal integer string=w374:string)  [unwired: 1 in]
                      n305 = Number To Decimal String(number=w363) -> (decimal integer string=w373:string)  [unwired: 1 in]
                      n306 = Number To Decimal String(number=w362) -> (decimal integer string=w372:string)  [unwired: 1 in]
                      n307 = Number To Decimal String(number=w355) -> (decimal integer string=w345:string)  [unwired: 1 in]
                      n308 = Number To Decimal String(number=w356) -> (decimal integer string=w346:string)  [unwired: 1 in]
                      n309 = Number To Decimal String(number=w357) -> (decimal integer string=w347:string)  [unwired: 1 in]
                      n310 = Number To Decimal String(number=w325) -> (decimal integer string=w333:string)  [unwired: 1 in]
                      n311 = Number To Decimal String(number=w324) -> (decimal integer string=w332:string)  [unwired: 1 in]
                      n312 = Number To Decimal String(number=w323) -> (decimal integer string=w319:string)  [unwired: 1 in]
                      n313 = Concatenate Strings(w461, w460, w459) -> (w458:string)
                      n314 = Concatenate Strings(w432, w433, w434) -> (w435:string)
                      n315 = Concatenate Strings(w418, w417, w416) -> (w415:string)
                      n316 = Concatenate Strings(w389, w390, w391) -> (w392:string)
                      n317 = Concatenate Strings(w374, w373, w372) -> (w371:string)
                      n318 = Concatenate Strings(w345, w346, w347) -> (w348:string)
                      n319 = Concatenate Strings(w333, w332, w319) -> (w331:string)
                      n320 = Decimal String To Number(string=w458) -> (number=w513:i32)  [unwired: 2 in, 1 out]
                      n321 = Decimal String To Number(string=w435) -> (number=w503:i32)  [unwired: 2 in, 1 out]
                      n322 = Decimal String To Number(string=w415) -> (number=w501:i32)  [unwired: 2 in, 1 out]
                      n323 = Decimal String To Number(string=w392) -> (number=w499:i32)  [unwired: 2 in, 1 out]
                      n324 = Decimal String To Number(string=w371) -> (number=w498:i32)  [unwired: 2 in, 1 out]
                      n325 = Decimal String To Number(string=w348) -> (number=w496:i32)  [unwired: 2 in, 1 out]
                      n326 = Decimal String To Number(string=w331) -> (number=w494:i32)  [unwired: 2 in, 1 out]
                      n327 = Multiply(x=w513, y=10) -> (x*y=w511:i32)
                      n328 = Divide(x=w503, y=100) -> (x/y=w504:dbl)
                      n329 = Divide(x=w501, y=100) -> (x/y=w502:dbl)
                      n330 = Divide(x=w499, y=100) -> (x/y=w500:dbl)
                      n331 = Divide(x=w498, y=100) -> (x/y=w497:dbl)
                      n332 = Divide(x=w496, y=100) -> (x/y=w495:dbl)
                      n333 = Divide(x=w494, y=100) -> (x/y=w493:dbl)
                      n334 = call "string_inteira_carater.vi"("String in"=w293) -> ("String out"=w492:string)  [unwired: 10 in]
                      n335 = local write "String lida em Caracter"(w492) -> ()
                    }
                    n336 = Build Array(w291, w285, w286, w287, w288, w289, w290) -> (w283:dbl[][])
                    n337 = Build Array (concatenate)(w283) -> (w280:T3)
                    "appended array" <- w280
                    n338 = Delete From Array(array=w280, index (row)=0) -> (array with subset deleted=w278:T3)  [unwired: 2 in, 1 out]
                    n339 = Bundle(0.0, 20.0, "Real Matrix"=w278) -> (→"Gráfico":cluster{dbl, dbl, "Real Matrix":T3})  [unwired: 1 in]
                  }
                }
              }
              frame #2 {
                n340 = flat-sequence {
                  frame #0 {
                    n341 = local write "MWU1100"(i16 200 ("MWU1100")) -> ()
                  }
                  frame #1 {
                    (unwired) "OK" ("button name (\"OK\")")
                    n342 = for {
                      N: 900 -> [_]
                      i -> [w530]
                      n343 = Multiply(x=w530, y=2.13) -> (x*y=w528:dbl)
                      n344 = Wait (ms)(milliseconds to wait=u32 100) -> ()  [unwired: 1 out]
                      n345 = Subtract(x=1920.0, y=w528) -> (x-y=w526:dbl)
                      n346 = local write "Tubo"(w526) -> ()
                    }
                    n347 = One Button Dialog(message="Sensor está retornando para HOME") -> ()  [unwired: 1 in, 1 out]
                  }
                  frame #2 {
                    n348 = while {
                      stop <- w532 stop-if-true
                      n349 = local read "MWU2975"() -> (w553:i16)
                      n350 = local read "MWU2976"() -> (w552:i16)
                      n351 = local read "MWU2977"() -> (w551:i16)
                      n352 = local read "MWU2978"() -> (w550:i16)
                      n353 = local read "MWU2979"() -> (w549:i16)
                      n354 = local read "MWU2980"() -> (w548:i16)
                      n355 = local read "MWU2981"() -> (w547:i16)
                      n356 = local read "MWU2982"() -> (w546:i16)
                      n357 = local read "MWU2983"() -> (w545:i16)
                      n358 = local read "MWU2984"() -> (w544:i16)
                      n359 = local read "MWU2985"() -> (w543:i16)
                      n360 = local read "MWU2986"() -> (w542:i16)
                      n361 = local read "MWU2987"() -> (w541:i16)
                      n362 = call "Conversor-bin-hex.vi"("Numeric"=w553) -> ("hex integer string"=w577:string)  [unwired: 9 in, 1 out]
                      n363 = call "Conversor-bin-hex.vi"("Numeric"=w552) -> ("hex integer string"=w575:string, "hex integer string 2"=w576:string)  [unwired: 9 in]
                      n364 = call "Conversor-bin-hex.vi"("Numeric"=w551) -> ("hex integer string"=w573:string, "hex integer string 2"=w574:string)  [unwired: 9 in]
                      n365 = call "Conversor-bin-hex.vi"("Numeric"=w550) -> ("hex integer string"=w571:string, "hex integer string 2"=w572:string)  [unwired: 9 in]
                      n366 = call "Conversor-bin-hex.vi"("Numeric"=w549) -> ("hex integer string"=w569:string, "hex integer string 2"=w570:string)  [unwired: 9 in]
                      n367 = call "Conversor-bin-hex.vi"("Numeric"=w548) -> ("hex integer string"=w567:string, "hex integer string 2"=w568:string)  [unwired: 9 in]
                      n368 = call "Conversor-bin-hex.vi"("Numeric"=w547) -> ("hex integer string"=w565:string, "hex integer string 2"=w566:string)  [unwired: 9 in]
                      n369 = call "Conversor-bin-hex.vi"("Numeric"=w546) -> ("hex integer string"=w563:string, "hex integer string 2"=w564:string)  [unwired: 9 in]
                      n370 = call "Conversor-bin-hex.vi"("Numeric"=w545) -> ("hex integer string"=w561:string, "hex integer string 2"=w562:string)  [unwired: 9 in]
                      n371 = call "Conversor-bin-hex.vi"("Numeric"=w544) -> ("hex integer string"=w559:string, "hex integer string 2"=w560:string)  [unwired: 9 in]
                      n372 = call "Conversor-bin-hex.vi"("Numeric"=w543) -> ("hex integer string"=w557:string, "hex integer string 2"=w558:string)  [unwired: 9 in]
                      n373 = call "Conversor-bin-hex.vi"("Numeric"=w542) -> ("hex integer string"=w555:string, "hex integer string 2"=w556:string)  [unwired: 9 in]
                      n374 = call "Conversor-bin-hex.vi"("Numeric"=w541) -> ("hex integer string"=w540:string, "hex integer string 2"=w554:string)  [unwired: 9 in]
                      n375 = Concatenate Strings(w577, w576, w575, w574, w573, w572, w571, w570, w569, w568, w567, w566, w565, w564, w563, w562, w561, w560, w559, w558, w557, w556, w555, w554, w540) -> (w539:string)
                      n376 = call "string_inteira_carater.vi"("String in"=w539) -> ("String out"=w538:string)  [unwired: 10 in]
                      n377 = local write "String lida em Caracter"(w538) -> ()
                      n378 = String Subset(string=w538, offset (0)=3, length (rest)=1 ("length (rest)")) -> (substring=w535:string)
                      n379 = Equal?(x="H", y=w535) -> (x = y?=w533:bool)
                      n380 = case shown="False" w533 {
                        tunnel: [FALSE TRUE] -> w532
                        frame False {
                          n381 = flat-sequence {
                            frame #0 {
                              n382 = local write "MWU1100"(i16 456 ("MWU1100")) -> ()
                            }
                            frame #1 {
                              n383 = Wait (ms)(milliseconds to wait=u32 250) -> ()  [unwired: 1 out]
                            }
                            frame #2 {
                              n384 = local write "MWU1100"(i16 200 ("MWU1100")) -> ()
                            }
                          }
                        }
                        frame True {
                        }
                      }
                    }
                  }
                  frame #3 {
                    n385 = local write "Iniciar"(FALSE ("Iniciar")) -> ()
                    n386 = property on="Parar" class="Bool (strict)"("DisabledEnum"=T2."Enabled" ("Disabled")) -> ()  [unwired: 2 in, 2 out]
                  }
                }
              }
            }
          }
          frame 2 {
          }
        }
      }
    }
  }
  n387 = property class="VI"(error in=w1, "Front Panel.Open"=FALSE ("Front Panel Window:Open")) -> ()  [unwired: 1 in, 2 out]
